vi "led_blink.vi"(8 "CurrentState":string, 11 "Action":enum16{"Entry", "During", "Exit"}(ring)) -> (0 "NextState":string)   [LabVIEW 2021]
uses:
  led_globals.vi
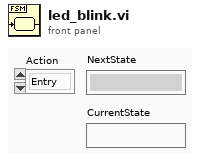
[diagram p1: front panel]
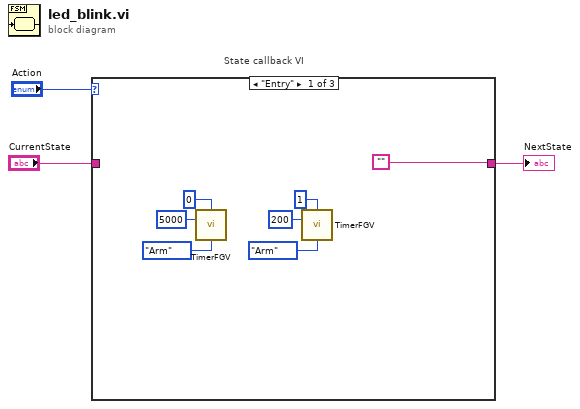
[diagram p0: block diagram]
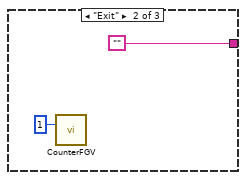
[diagram p2: hidden frame]
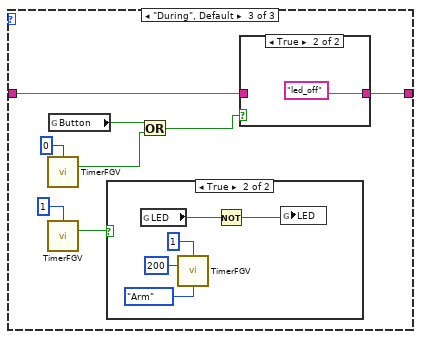
[diagram p3: hidden frame]
diagram:
  # "State callback VI"
  n1 = case shown="\"Entry\"" "Action" {
    tunnel: ["" "" w20] -> w2
    tunnel: "CurrentState" -> [_ _ w19]
    frame "Entry" {
      n2 = call "TimerFGV.vi"("index"=0, "time(ms)"=u32 5000, "action"=enum16{"Check", "Arm", "Disarm", "Init"}."Arm") -> ()  [unwired: 10 in, 3 out]
      n3 = call "TimerFGV.vi"("index"=1, "time(ms)"=u32 200, "action"=enum16{"Check", "Arm", "Disarm", "Init"}."Arm") -> ()  [unwired: 10 in, 3 out]
    }
    frame "Exit" {
      n4 = call "CounterFGV.vi"("val/inc"=1) -> ()  [unwired: 13 in, 2 out]
    }
    frame "During", Default {
      n5 = call "TimerFGV.vi"("index"=0) -> ("expired?"=w15:bool)  [unwired: 12 in, 2 out]
      n6 = call "TimerFGV.vi"("index"=1) -> ("expired?"=w13:bool)  [unwired: 12 in, 2 out]
      n7 = global read "led_globals.vi" "Button"() -> (w18:bool)
      n8 = case shown="True" w13 {
        frame False {
        }
        frame True {
          n9 = global read "led_globals.vi" "LED"() -> (w22:bool)
          n10 = call "TimerFGV.vi"("index"=1, "time(ms)"=u32 200, "action"=enum16{"Check", "Arm", "Disarm", "Init"}."Arm") -> ()  [unwired: 10 in, 3 out]
          n11 = Not(x=w22) -> (.not. x?=w21:bool)
          n12 = global write "led_globals.vi" "LED"(w21) -> ()
        }
      }
      n13 = Or(x=w18, y=w15) -> (x .or. y?=w17:bool)
      n14 = case shown="True" w17 {
        tunnel: [w26 "led_off"] -> w20
        tunnel: w19 -> [w26 _]
        frame False {
        }
        frame True {
        }
      }
    }
  }
  "NextState" <- w2
